vi "PUERTOS USART.vi"(0 "VISA resource name":refnum<visa-resource-name>, 5 "PUERTO":u8(ring) items=["USART"], 7 "OPERACION":u8(ring) items=["SALIDA", "ENTRADA"], 9 "DATO":u8 step=255, 11 "error":errorcluster, 12 "HABILITA":bool) -> (4 "VISA resource name":refnum<visa-resource-name>, 6 "RESULTADO":string, 8 "Resultado U8":u8, 15 "error":errorcluster)   [LabVIEW 2009]
panel:
  out "return count":u32
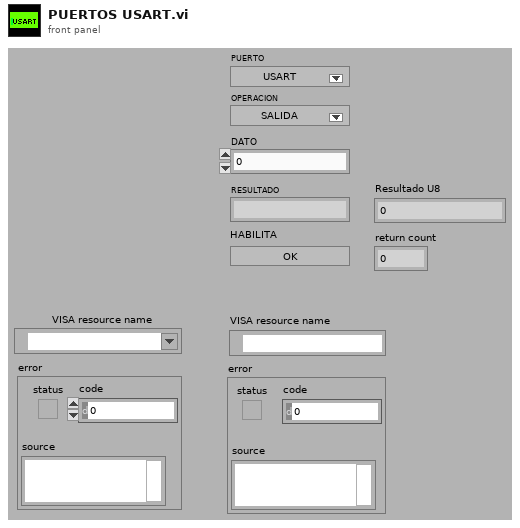
[diagram p1: front panel]
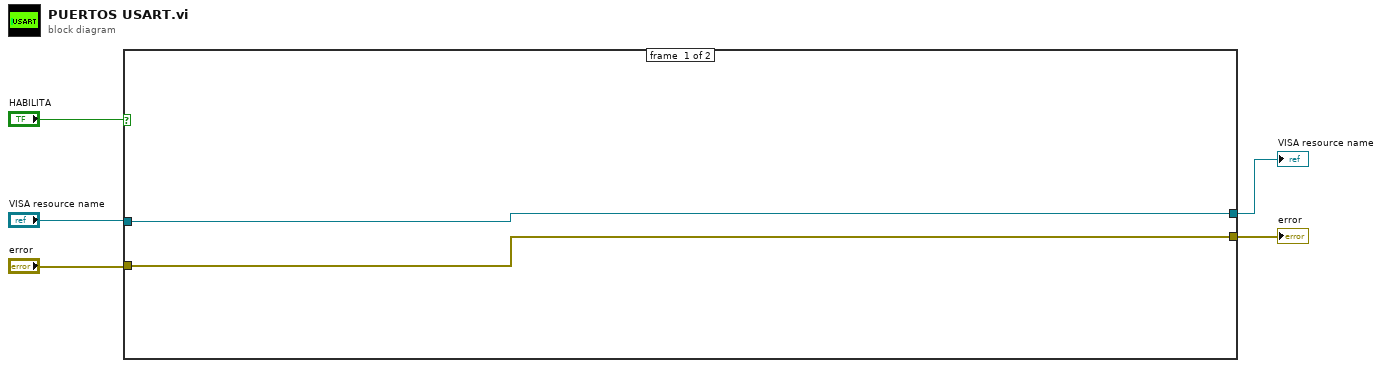
[diagram p0: block diagram]
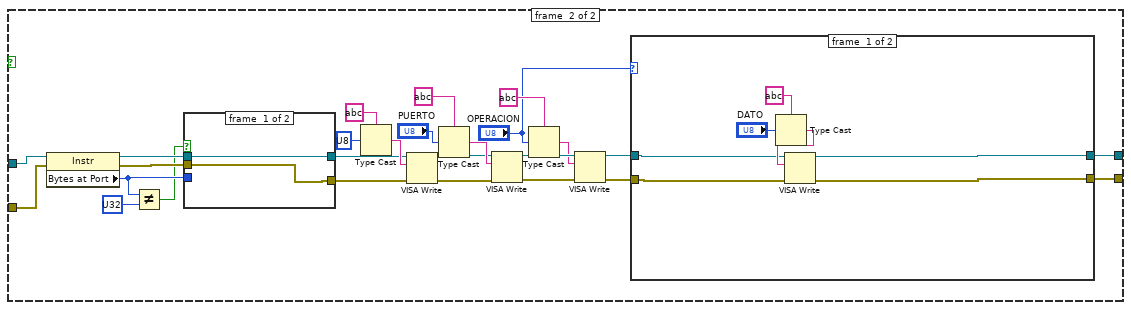
[diagram p2: hidden frame]
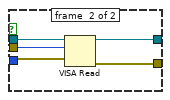
[diagram p3: hidden frame]
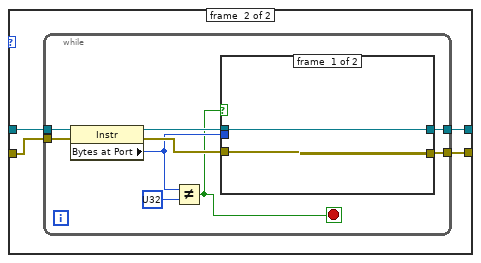
[diagram p4: hidden frame]
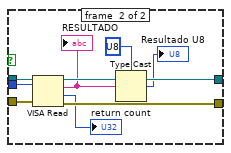
[diagram p5: hidden frame]
diagram:
  n1 = case shown="True" "HABILITA" {
    tunnel: "VISA resource name" -> [w7 w11]
    tunnel: "error" -> [w6 w8]
    tunnel: [w7 w26] -> w3
    tunnel: [w6 w33] -> w2
    frame #0 {
    }
    frame #1 {
      n2 = property class="Instr"(reference=w11, error in=w8) -> (reference out=w16:refnum<visa-resource-name>, error out=w15:errorcluster, "Bytes at Port"=w14:u32)
      n3 = Not Equal?(x=w14, y=u32 ?) -> (x != y?=w12:bool)
      n4 = case shown="True" w12 {
        tunnel: w16 -> [w35 w40]
        tunnel: w15 -> [w34 w39]
        tunnel: w14 -> [_ w38]
        tunnel: [w35 w37] -> w10
        tunnel: [w34 w36] -> w9
        frame #0 {
        }
        frame #1 {
          n5 = VISA Read(VISA resource name=w40, byte count=w38, error in (no error)=w39) -> (VISA resource name out=w37:refnum<visa-resource-name>, error out=w36:errorcluster)  [unwired: 2 out]
        }
      }
      n6 = Type Cast(type=string ?, x=u8 ?) -> (*(type *) &x=w24:string)
      n7 = VISA Write(VISA resource name=w10, write buffer=w24, error in (no error)=w9) -> (VISA resource name out=w21:refnum<visa-resource-name>, error out=w23:errorcluster)  [unwired: 1 out]
      n8 = Type Cast(type=string ?, x="PUERTO") -> (*(type *) &x=w29:string)
      n9 = VISA Write(VISA resource name=w21, write buffer=w29, error in (no error)=w23) -> (VISA resource name out=w32:refnum<visa-resource-name>, error out=w22:errorcluster)  [unwired: 1 out]
      n10 = Type Cast(type=string ?, x="OPERACION") -> (*(type *) &x=w27:string)
      n11 = VISA Write(VISA resource name=w32, write buffer=w27, error in (no error)=w22) -> (VISA resource name out=w19:refnum<visa-resource-name>, error out=w18:errorcluster)  [unwired: 1 out]
      n12 = case shown="1" "OPERACION" {
        tunnel: [w41 w51] -> w33
        tunnel: w19 -> [w44 w50]
        tunnel: w18 -> [w43 w49]
        tunnel: [w42 w48] -> w26
        frame #0 {
          n13 = Type Cast(type=string ?, x="DATO") -> (*(type *) &x=w47:string)
          n14 = VISA Write(VISA resource name=w44, write buffer=w47, error in (no error)=w43) -> (VISA resource name out=w42:refnum<visa-resource-name>, error out=w41:errorcluster)  [unwired: 1 out]
        }
        frame #1 {
          n15 = while {
            tunnel: [w52] -> w48
            tunnel: [w60] -> w51
            tunnel: w50 -> [w59]
            tunnel: w49 -> [w56]
            stop <- w53 stop-if-true
            n16 = property class="Instr"(reference=w59, error in=w56) -> (reference out=w58:refnum<visa-resource-name>, error out=w57:errorcluster, "Bytes at Port"=w55:u32)
            n17 = Not Equal?(x=w55, y=u32 ?) -> (x != y?=w53:bool)
            n18 = case shown="True" w53 {
              tunnel: [w62 w67] -> w52
              tunnel: [w61 w71] -> w60
              tunnel: w58 -> [w62 w70]
              tunnel: w57 -> [w61 w69]
              tunnel: w55 -> [_ w68]
              frame #0 {
              }
              frame #1 {
                n19 = VISA Read(VISA resource name=w70, byte count=w68, error in (no error)=w69) -> (VISA resource name out=w67:refnum<visa-resource-name>, read buffer=w66:string, return count=→"return count":u32, error out=w71:errorcluster)
                "RESULTADO" <- w66
                n20 = Type Cast(type=u8 ?, x=w66) -> (*(type *) &x=→"Resultado U8":u8)
              }
            }
          }
        }
      }
    }
  }
  "VISA resource name" <- w3
  "error" <- w2
